vi "Kasir.vi"() -> ()   [LabVIEW 2022 SP3]
panel:
  in  "Bayar":bool
  out "Kembalian":dbl
  in  "Jumlah Uang":dbl
  in  "Konfirmasi":bool
  out "Discount":string
  out "Total Harga":dbl
  out "Harga 4":dbl
  in  "Jumlah 4":dbl=1.0 min=0.0 max=10.0
  in  "Teh Manis":bool
  out "Harga 3":dbl
  in  "Jumlah 3":dbl=1.0 min=0.0 max=10.0
  in  "Nasi Goreng":bool
  out "Harga 2":dbl
  in  "Jumlah 2":dbl=1.0 min=0.0 max=10.0
  in  "Ayam Goreng":bool
  out "Harga":dbl
  in  "Jumlah":dbl=1.0 min=0.0 max=10.0
  in  "Pisang Goreng":bool
  # "KANTIN POLMAN BANDUNG"
  # "#"
  # "Harga"
  # "Menu"
  # "Jumlah"
  # "Pisang Goreng"
  # "Ayam Goreng"
  # "Nasi Goreng"
  # "Teh Manis"
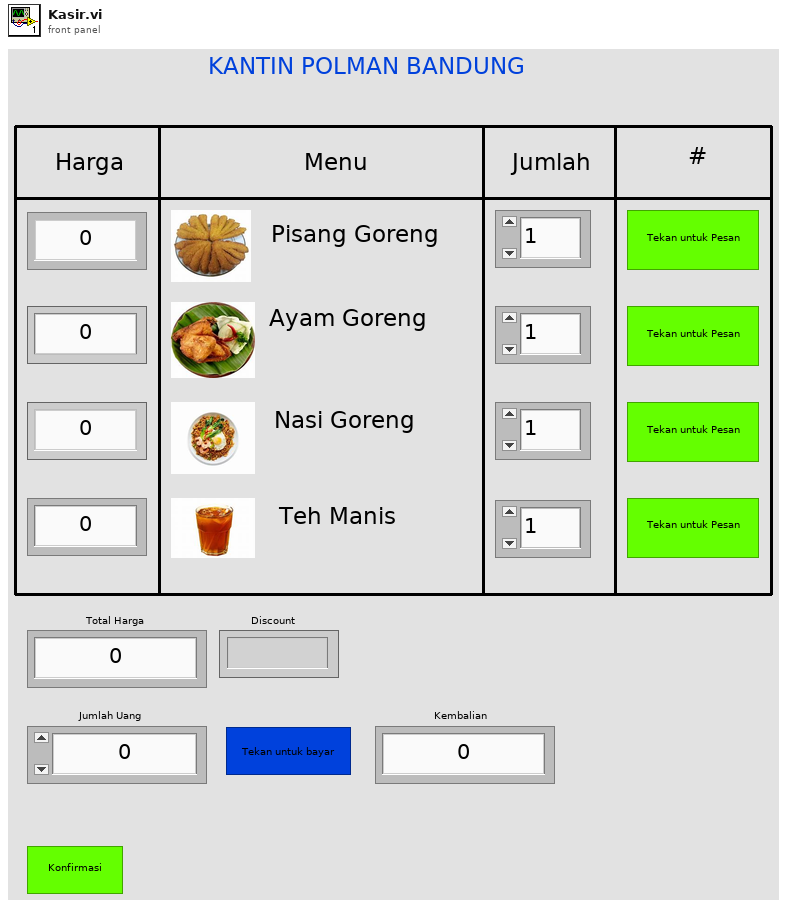
[diagram p1: front panel]
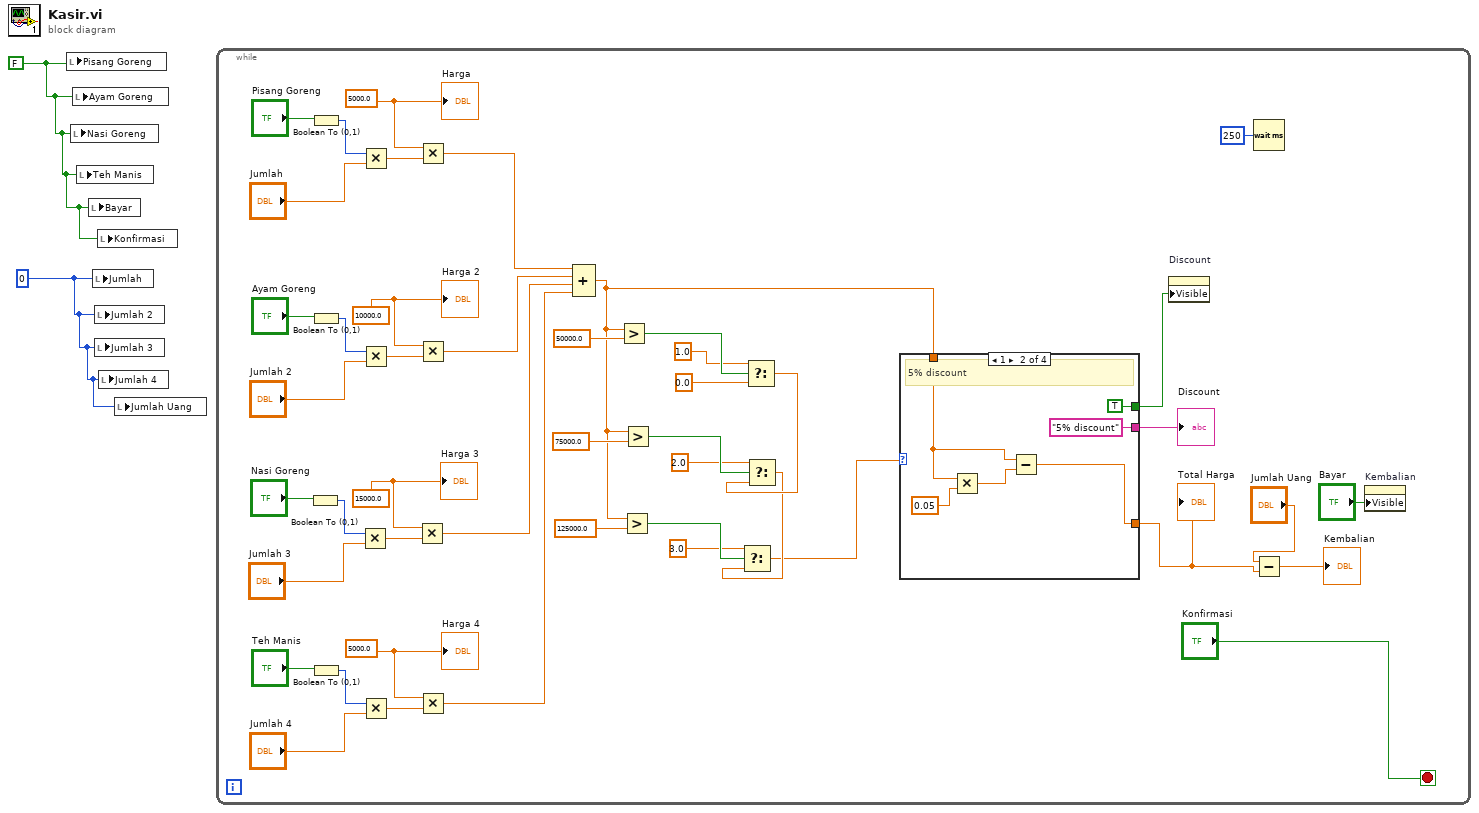
[diagram p0: block diagram]
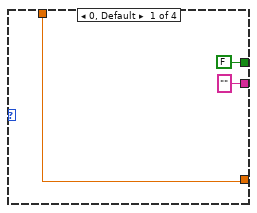
[diagram p2: hidden frame]
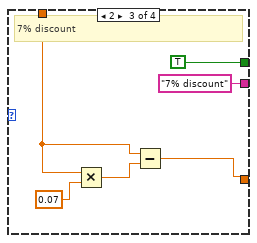
[diagram p3: hidden frame]
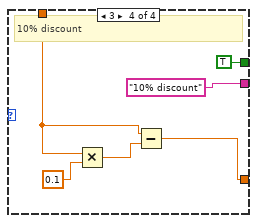
[diagram p4: hidden frame]
diagram:
  w2 = 0
  w1 = FALSE ("Paket HTS")
  n1 = local write "Pisang Goreng"(w1) -> ()
  n2 = local write "Nasi Goreng"(w1) -> ()
  n3 = local write "Ayam Goreng"(w1) -> ()
  n4 = local write "Teh Manis"(w1) -> ()
  n5 = local write "Bayar"(w1) -> ()
  n6 = local write "Jumlah"(w2) -> ()
  n7 = local write "Jumlah 2"(w2) -> ()
  n8 = local write "Jumlah 3"(w2) -> ()
  n9 = local write "Konfirmasi"(w1) -> ()
  n10 = local write "Jumlah 4"(w2) -> ()
  n11 = local write "Jumlah Uang"(w2) -> ()
  n12 = while {
    stop <- "Konfirmasi" stop-if-true
    w29 = 5000.0 ("Harga")
    w34 = 15000.0 ("Harga")
    w39 = 10000.0 ("Harga")
    w44 = 5000.0 ("Harga")
    n13 = Boolean To (0,1)(Boolean="Nasi Goreng") -> (0, 1=w37:i16)
    n14 = Boolean To (0,1)(Boolean="Pisang Goreng") -> (0, 1=w47:i16)
    n15 = Boolean To (0,1)(Boolean="Ayam Goreng") -> (0, 1=w42:i16)
    n16 = Boolean To (0,1)(Boolean="Teh Manis") -> (0, 1=w32:i16)
    n17 = Multiply(x=w37, y="Jumlah 3") -> (x*y=w35:dbl)
    n18 = Multiply(x=w47, y="Jumlah") -> (x*y=w45:dbl)
    n19 = Multiply(x=w42, y="Jumlah 2") -> (x*y=w40:dbl)
    n20 = Multiply(x=w32, y="Jumlah 4") -> (x*y=w30:dbl)
    n21 = Multiply(x=w34, y=w35) -> (x*y=w26:dbl)
    n22 = Multiply(x=w44, y=w45) -> (x*y=w28:dbl)
    n23 = Multiply(x=w39, y=w40) -> (x*y=w27:dbl)
    n24 = Multiply(x=w29, y=w30) -> (x*y=w25:dbl)
    n25 = Compound Arithmetic op=ADD(w28, w27, w26, w25) -> (w11:dbl)
    n26 = Greater?(x=w11, y=50000.0) -> (0:w21:bool)
    n27 = Greater?(x=w11, y=125000.0) -> (0:w15:bool)
    n28 = Greater?(x=w11, y=75000.0) -> (0:w18:bool)
    n29 = Select(t=1.0, s=w21, f=0.0) -> (s? t:f=w16:dbl)
    n30 = Select(t=2.0, s=w18, f=w16) -> (s? t:f=w13:dbl)
    n31 = Select(t=3.0, s=w15, f=w13) -> (s? t:f=w12:dbl)
    n32 = case shown="1" w12 {
      tunnel: w11 -> [w51 w56 w61 w67]
      tunnel: [w51 w54 w60 w66] -> w6
      tunnel: ["" ("Discount") "5% discount" ("Discount") "7% discount" ("Discount") "10% discount" ("Discount")] -> w10
      tunnel: [FALSE ("Visible") TRUE ("Visible") TRUE ("Visible") TRUE ("Visible")] -> w9
      frame 0, Default {
      }
      frame 1 {
        # "5% discount"
        n33 = Multiply(x=w56, y=0.05) -> (x*y=w55:dbl)
        n34 = Subtract(x=w56, y=w55) -> (x-y=w54:dbl)
      }
      frame 2 {
        # "7% discount"
        n35 = Multiply(x=w61, y=0.07) -> (x*y=w63:dbl)
        n36 = Subtract(x=w61, y=w63) -> (x-y=w60:dbl)
      }
      frame 3 {
        # "10% discount"
        n37 = Multiply(x=w67, y=0.1) -> (x*y=w69:dbl)
        n38 = Subtract(x=w67, y=w69) -> (x-y=w66:dbl)
      }
    }
    "Total Harga" <- w6
    "Discount" <- w10
    n39 = property on="Discount" class="Str"("Visible"=w9) -> ()  [unwired: 2 in, 2 out]
    n40 = Wait (ms)(milliseconds to wait=u32 250) -> ()  [unwired: 1 out]
    n41 = Subtract(x="Jumlah Uang", y=w6) -> (x-y=→"Kembalian":dbl)
    n42 = property on="Kembalian" class="DigNum (strict)"("Visible"="Bayar") -> ()  [unwired: 2 in, 2 out]
    "Harga" <- w44
    "Harga 2" <- w39
    "Harga 3" <- w34
    "Harga 4" <- w29
  }
